vi "Get TX Message.vi"(8 "error in (no error)":errorcluster, 11 "RxTx in":refnum<class "RxTx.lvclass">) -> (0 "error out":errorcluster, 2 "New msg":bool, 3 "RxTx out":refnum<class "RxTx.lvclass">)   [LabVIEW 2018, in "RxTx.lvclass"]
doc: "Pop the lastest Tx message found in the qeue"
uses:
  RxTx.lvclass
  RxTx.lvclass/RxTx.ctl
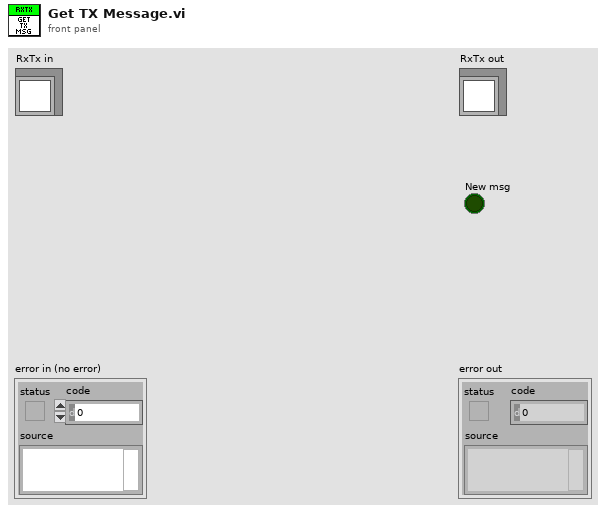
[diagram p1: front panel]
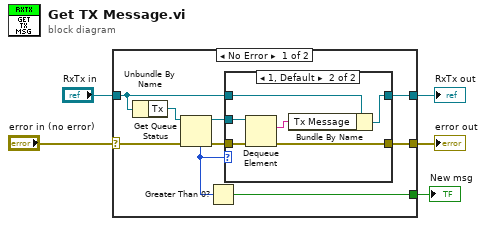
[diagram p0: block diagram]
diagram:
  n1 = case shown="No Error" "error in (no error)" {
    selector: "error in (no error)" -> [w11 w24]
    tunnel: [w9 w24] -> w3
    tunnel: [w13 w23] -> w2
    tunnel: "RxTx in" -> [w14 w23]
    tunnel: [w6 _] -> w1
    frame No Error {
      n2 = Unbundle By Name(w14) -> ("Tx"=w12:refnum<queue>)
      n3 = Get Queue Status(queue=w12, error in (no error)=w11) -> (queue out=w8:refnum<queue>, error out=w10:errorcluster, # elements in queue=w7:i32)  [unwired: 1 in, 5 out]
      n4 = Greater Than 0?(x=w7) -> (x > 0?=w6:bool)
      n5 = case shown="1, Default" w7 {
        tunnel: w14 -> [w15 w22]
        tunnel: [w15 w21] -> w13
        tunnel: w10 -> [w16 w19]
        tunnel: [w16 w18] -> w9
        tunnel: w8 -> [_ w17]
        frame 0 {
        }
        frame 1, Default {
          n6 = Dequeue Element(queue=w17, error in (no error)=w19) -> (element=w20:string, error out=w18:errorcluster)  [unwired: 1 in, 2 out]
          n7 = Bundle By Name(cluster=w22, "Tx Message"=w20) -> (w21:refnum<class "RxTx.lvclass">)
        }
      }
    }
    frame Error {
    }
  }
  "error out" <- w3
  "RxTx out" <- w2
  "New msg" <- w1
